vi "Get Param.vi"(8 "error in (no error)":errorcluster, 11 "paramID":i32) -> (0 "error out":errorcluster, 2 "param out":dbl, 3 "function return":i32)   [LabVIEW 2020, in "ThorECU.lvlib"]
doc: "long GetParam(const long paramID, double &param);"
uses:
  ThorECU.lvlib
  ThorECU.dll
panel:
  in  "param":dbl
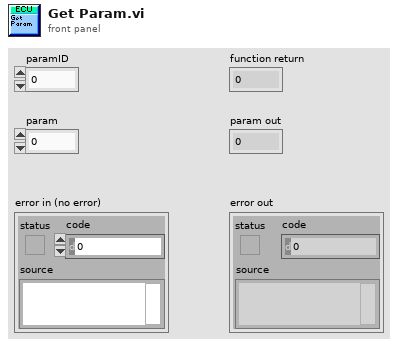
[diagram p1: front panel]
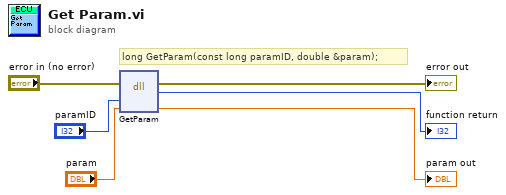
[diagram p0: block diagram]
diagram:
  # "long GetParam(const long paramID, double &param);"
  n1 = dll-call lib="D:/software/TweezerTron/ThorECU.*" fn="GetParam"(error in="error in (no error)", "paramID"="paramID", "param"="param") -> (error out=→"error out":errorcluster, "return type"=→"function return":i32, "param"=→"param out":dbl)  [unwired: 3 in, 1 out]
